vi "CRYUnflatten Stimulus.vi"(11 "Flatten Stimulus":string) -> (0 "Error?":bool=TRUE, 2 "Stimulus":T1={"StimulusType"="", "UseMLValArray"=[], "ML_axisArray"=[], "MLValLevelNameArray"=[], "Level(U)Array"=[1.0, 0.0, 0.0, 0.0, 0.0, 0.0, 0.26], "Start(Stop)FreqArray"=[20000.0, 20.0], "Start(Stop)AmpArray"=[0.5, 1.0], "StepResolutionArray"=[], "Unit_Array"=[], "DegValArray"=[], "DegUnitArray"=[], "Steps1"=19, "Cycle/step1(#)"=20, "Time/step1(s)"=0.01, "Transition1"=0.0, "SweepRate2"=1.0, "Freq3(Hz)"=0.0, "Steps3(#)"=19.0, "Cycles3(#)"=12, "StepSize3"=0.0, "wave time"="", "RMS_Value4"=0.0, "Peak_Value4"=0.0, "WavePath4"="", "RMS_unit4"="", "Peak_unit4"="", "wave Info"="", "dc_ctrl5_1"=0, "dc_ctrl5_2"=0, "dc_polar5"=0, "Max.Current"=0, "Steps5(#)"=19, "Time/Step5"=0.05, "Level5"=0.0, "StepsSize5Val"=0.0, "StepSize5Unit"="", "SweepType"=0, "Fixed/Ratio6"=0, "Transition6"=0.0, "Steps6(#)"=19.0, "Cycle/Steps6(#)"=12, "Time/Steps6(s)"=0.0, "Freq6(Hz)"=0.0, "Difference6(Hz)"=0.0, "Ratio6"="", "NoiseType7"=0, "Duration7(s)"=1.0, "MinFreq7(Hz)"=20000.0, "MaxFreq7(Hz)"=20.0, "MinFreq8(Hz)"=20000.0, "MaxFreq8(Hz)"=20.0, "FreqRounding8"=FALSE, "Duration8(s)"=1.0, "Tones8"=0.0, "RoundingVal8"=0.0, "ApplyEQ"=FALSE, "Duration(s)"=0.0, "CustomStimulusName "="", "Flatten Element Array"=[], "sine waves"=[], "Channel Out"=0, "RatioVal6"=0.0, "TabCtrl6"=enum."Master Tone", "Signal Type Name"="", "Help"="", "Channel Sel"=19, "V on DUT"=FALSE, "Output Imp"=6300.0, "Nominal Imp"=100.0} {"Nominal Imp" format="%.2p"; "Output Imp" format="%.2p"; "sine waves"."cycles" format="%.2f"; "sine waves"."ampl" format="%.2f"; "sine waves"."freq" format="%.2f"}, 3 "Header info":T2={"Data type"="Data            ", "Version"=1, "Dimensions"=0})   [LabVIEW 2013]
uses:
  Typedef Control/CRYStimulus Cluster.ctl
panel:
  # "(1,2,3,4,6_1,6_2,7,8)"
  # "(1,2,3,4,6_1,6_2,7,8)"
  # "(1,2,3,4,6_1,6_2,7,8)"
  # "(1,2,4,6_1,6_2,7,8)"
  # "(1,2,6)"
  # "(3,5)"
  # "(1,6,8)"
  # "(1,2,4,6_1,6_2,7,8)"
  # "(1,2,3,4,6_1,6_2,7,8)"
  # "(1,2,3,4,6_1,6_2,7,8)"
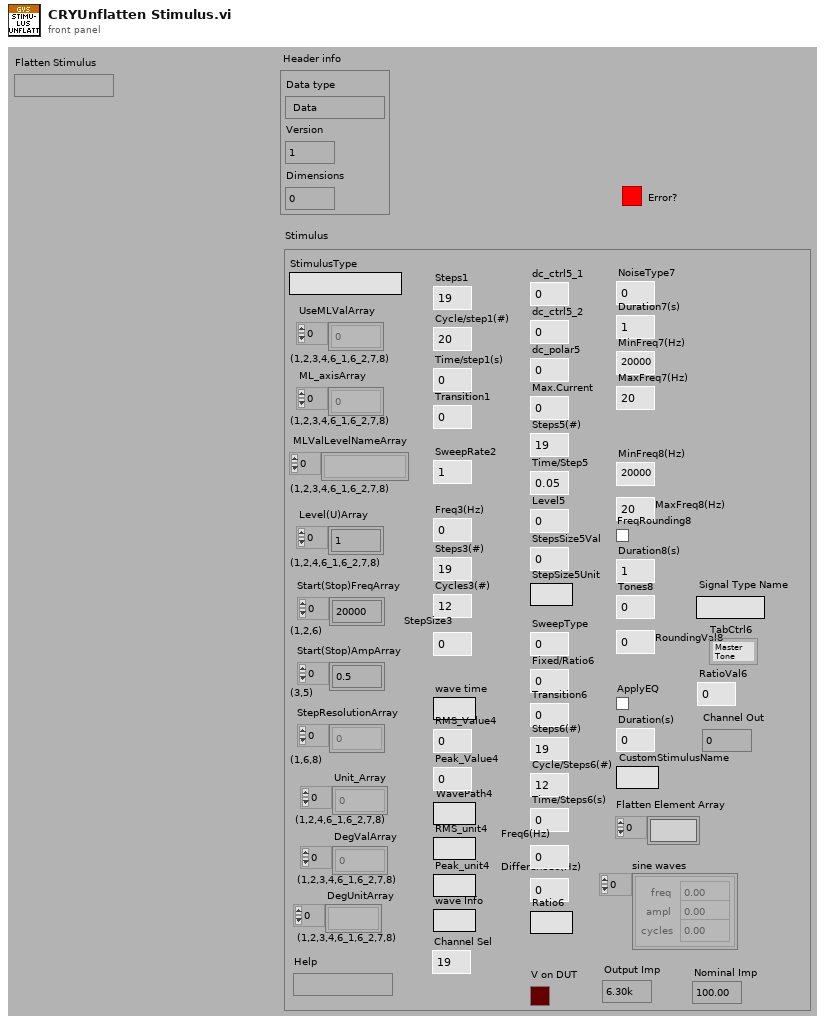
[diagram p1: front panel]
types:
  T1 = typedef "CRYStimulus Cluster.ctl" = cluster{"StimulusType":string, "UseMLValArray":u16[], "ML_axisArray":u16[], "MLValLevelNameArray":string[], "Level(U)Array":dbl[], "Start(Stop)FreqArray":dbl[], "Start(Stop)AmpArray":dbl[], "StepResolutionArray":u16[], "Unit_Array":u16[], "DegValArray":dbl[], "DegUnitArray":string[], "Steps1":i32, "Cycle/step1(#)":u32, "Time/step1(s)":dbl, "Transition1":dbl, "SweepRate2":dbl, "Freq3(Hz)":dbl, "Steps3(#)":dbl, "Cycles3(#)":u32, "StepSize3":dbl, "wave time":string, "RMS_Value4":dbl, "Peak_Value4":dbl, "WavePath4":string, "RMS_unit4":string, "Peak_unit4":string, "wave Info":string, "dc_ctrl5_1":u16, "dc_ctrl5_2":u16, "dc_polar5":u16, "Max.Current":u16, "Steps5(#)":u32, "Time/Step5":dbl, "Level5":dbl, "StepsSize5Val":dbl, "StepSize5Unit":string, "SweepType":u16, "Fixed/Ratio6":u16, "Transition6":dbl, "Steps6(#)":dbl, "Cycle/Steps6(#)":u32, "Time/Steps6(s)":dbl, "Freq6(Hz)":dbl, "Difference6(Hz)":dbl, "Ratio6":string, "NoiseType7":u16, "Duration7(s)":dbl, "MinFreq7(Hz)":dbl, "MaxFreq7(Hz)":dbl, "MinFreq8(Hz)":dbl, "MaxFreq8(Hz)":dbl, "FreqRounding8":bool, "Duration8(s)":dbl, "Tones8":dbl, "RoundingVal8":dbl, "ApplyEQ":bool, "Duration(s)":dbl, "CustomStimulusName ":string, "Flatten Element Array":string[], "sine waves":cluster{"freq":dbl, "ampl":dbl, "cycles":dbl}[], "Channel Out":i32, "RatioVal6":dbl, "TabCtrl6":enum32{"Master Tone", "Slave Tone"}, "Signal Type Name":string, "Help":string, "Channel Sel":u16, "V on DUT":bool, "Output Imp":dbl, "Nominal Imp":dbl}
  T2 = cluster{"Data type":string, "Version":u16, "Dimensions":u8}
  T3 = cluster{"unsigned byte array[0]":u8, "unsigned byte array[1]":u8, "unsigned byte array[2]":u8}
  T4 = cluster{"StimulusType":string, "UseMLValArray":u16[], "ML_axisArray":u16[], "MLValLevelNameArray":string[], "Level(U)Array":dbl[], "Start(Stop)FreqArray":dbl[], "Start(Stop)AmpArray":dbl[], "StepResolutionArray":string[], "Unit_Array":string[], "DegValArray":dbl[], "DegUnitArray":string[], "Steps1":i32, "Cycle/step1(#)":u32, "Time/step1(s)":dbl, "Transition1":dbl, "SweepRate2":dbl, "Freq3(Hz)":dbl, "Steps3(#)":dbl, "Cycles3(#)":u32, "StepSize3":dbl, "wave time":string, "RMS_Value4":dbl, "Peak_Value4":dbl, "WavePath4":string, "RMS_unit4":string, "Peak_unit4":string, "wave Info":string, "dc_ctrl5_1":u16, "dc_ctrl5_2":u16, "dc_polar5":u16, "Max.Current":u16, "Steps5(#)":u32, "Time/Step5":dbl, "Level5":dbl, "StepsSize5Val":dbl, "StepSize5Unit":string, "SweepType":u16, "Fixed/Ratio6":u16, "Transition6":dbl, "Steps6(#)":dbl, "Cycle/Steps6(#)":u32, "Time/Steps6(s)":dbl, "Freq6(Hz)":dbl, "Difference6(Hz)":dbl, "Ratio6":string, "NoiseType7":u16, "Duration7(s)":dbl, "MinFreq7(Hz)":dbl, "MaxFreq7(Hz)":dbl, "MinFreq8(Hz)":dbl, "MaxFreq8(Hz)":dbl, "FreqRounding8":bool, "Duration8(s)":dbl, "Tones8":dbl, "RoundingVal8":dbl, "ApplyEQ":bool, "Duration(s)":dbl, "CustomStimulusName ":string, "Flatten Element Array":string[], "sine waves":cluster{"freq":dbl, "ampl":dbl, "cycles":dbl}[], "Channel In":i32, "RatioVal6":dbl, "TabCtrl6":enum32{"Master Tone", "Slave Tone"}, "Channel Name":string}
  T5 = cluster{"StimulusType":string, "UseMLValArray":u16[], "ML_axisArray":u16[], "MLValLevelNameArray":string[], "Level(U)Array":dbl[], "Start(Stop)FreqArray":dbl[], "Start(Stop)AmpArray":dbl[], "StepResolutionArray":u16[], "Unit_Array":u16[], "DegValArray":dbl[], "DegUnitArray":string[], "Steps1":i32, "Cycle/step1(#)":u32, "Time/step1(s)":dbl, "Transition1":dbl, "SweepRate2":dbl, "Freq3(Hz)":dbl, "Steps3(#)":dbl, "Cycles3(#)":u32, "StepSize3":dbl, "wave time":string, "RMS_Value4":dbl, "Peak_Value4":dbl, "WavePath4":string, "RMS_unit4":string, "Peak_unit4":string, "wave Info":string, "dc_ctrl5_1":u16, "dc_ctrl5_2":u16, "dc_polar5":u16, "Max.Current":u16, "Steps5(#)":u32, "Time/Step5":dbl, "Level5":dbl, "StepsSize5Val":dbl, "StepSize5Unit":string, "SweepType":u16, "Fixed/Ratio6":u16, "Transition6":dbl, "Steps6(#)":dbl, "Cycle/Steps6(#)":u32, "Time/Steps6(s)":dbl, "Freq6(Hz)":dbl, "Difference6(Hz)":dbl, "Ratio6":string, "NoiseType7":u16, "Duration7(s)":dbl, "MinFreq7(Hz)":dbl, "MaxFreq7(Hz)":dbl, "MinFreq8(Hz)":dbl, "MaxFreq8(Hz)":dbl, "FreqRounding8":bool, "Duration8(s)":dbl, "Tones8":dbl, "RoundingVal8":dbl, "ApplyEQ":bool, "Duration(s)":dbl, "CustomStimulusName ":string, "Flatten Element Array":string[], "sine waves":cluster{"freq":dbl, "ampl":dbl, "cycles":dbl}[], "Channel In":i32, "RatioVal6":dbl, "TabCtrl6":enum32{"Master Tone", "Slave Tone"}, "Channel Name":string}
  T6 = cluster{"StimulusType":string, "UseMLValArray":u16[], "ML_axisArray":u16[], "MLValLevelNameArray":string[], "Level(U)Array":dbl[], "Start(Stop)FreqArray":dbl[], "Start(Stop)AmpArray":dbl[], "StepResolutionArray":u16[], "Unit_Array":u16[], "DegValArray":dbl[], "DegUnitArray":string[], "Steps1":i32, "Cycle/step1(#)":u32, "Time/step1(s)":dbl, "Transition1":dbl, "SweepRate2":dbl, "Freq3(Hz)":dbl, "Steps3(#)":dbl, "Cycles3(#)":u32, "StepSize3":dbl, "wave time":string, "RMS_Value4":dbl, "Peak_Value4":dbl, "WavePath4":string, "RMS_unit4":string, "Peak_unit4":string, "wave Info":string, "dc_ctrl5_1":u16, "dc_ctrl5_2":u16, "dc_polar5":u16, "Max.Current":u16, "Steps5(#)":u32, "Time/Step5":dbl, "Level5":dbl, "StepsSize5Val":dbl, "StepSize5Unit":string, "SweepType":u16, "Fixed/Ratio6":u16, "Transition6":dbl, "Steps6(#)":dbl, "Cycle/Steps6(#)":u32, "Time/Steps6(s)":dbl, "Freq6(Hz)":dbl, "Difference6(Hz)":dbl, "Ratio6":string, "NoiseType7":u16, "Duration7(s)":dbl, "MinFreq7(Hz)":dbl, "MaxFreq7(Hz)":dbl, "MinFreq8(Hz)":dbl, "MaxFreq8(Hz)":dbl, "FreqRounding8":bool, "Duration8(s)":dbl, "Tones8":dbl, "RoundingVal8":dbl, "ApplyEQ":bool, "Duration(s)":dbl, "CustomStimulusName ":string, "Flatten Element Array":string[], "sine waves":cluster{"freq":dbl, "ampl":dbl, "cycles":dbl}[], "Channel In":i32, "RatioVal6":dbl, "TabCtrl6":enum32{"Master Tone", "Slave Tone"}, "Channel Name":string, "Help":string}
  T7 = cluster{"StimulusType":string, "UseMLValArray":u16[], "ML_axisArray":u16[], "MLValLevelNameArray":string[], "Level(U)Array":dbl[], "Start(Stop)FreqArray":dbl[], "Start(Stop)AmpArray":dbl[], "StepResolutionArray":u16[], "Unit_Array":u16[], "DegValArray":dbl[], "DegUnitArray":string[], "Steps1":i32, "Cycle/step1(#)":u32, "Time/step1(s)":dbl, "Transition1":dbl, "SweepRate2":dbl, "Freq3(Hz)":dbl, "Steps3(#)":dbl, "Cycles3(#)":u32, "StepSize3":dbl, "wave time":string, "RMS_Value4":dbl, "Peak_Value4":dbl, "WavePath4":string, "RMS_unit4":string, "Peak_unit4":string, "wave Info":string, "dc_ctrl5_1":u16, "dc_ctrl5_2":u16, "dc_polar5":u16, "Max.Current":u16, "Steps5(#)":u32, "Time/Step5":dbl, "Level5":dbl, "StepsSize5Val":dbl, "StepSize5Unit":string, "SweepType":u16, "Fixed/Ratio6":u16, "Transition6":dbl, "Steps6(#)":dbl, "Cycle/Steps6(#)":u32, "Time/Steps6(s)":dbl, "Freq6(Hz)":dbl, "Difference6(Hz)":dbl, "Ratio6":string, "NoiseType7":u16, "Duration7(s)":dbl, "MinFreq7(Hz)":dbl, "MaxFreq7(Hz)":dbl, "MinFreq8(Hz)":dbl, "MaxFreq8(Hz)":dbl, "FreqRounding8":bool, "Duration8(s)":dbl, "Tones8":dbl, "RoundingVal8":dbl, "ApplyEQ":bool, "Duration(s)":dbl, "CustomStimulusName ":string, "Flatten Element Array":string[], "sine waves":cluster{"freq":dbl, "ampl":dbl, "cycles":dbl}[], "Channel Out":i32, "RatioVal6":dbl, "TabCtrl6":enum32{"Master Tone", "Slave Tone"}, "Signal Type Name":string, "Help":string, "Channel Sel":u16}
  T8 = cluster{"substring":string, u16, "unsigned byte array[2]":u8}
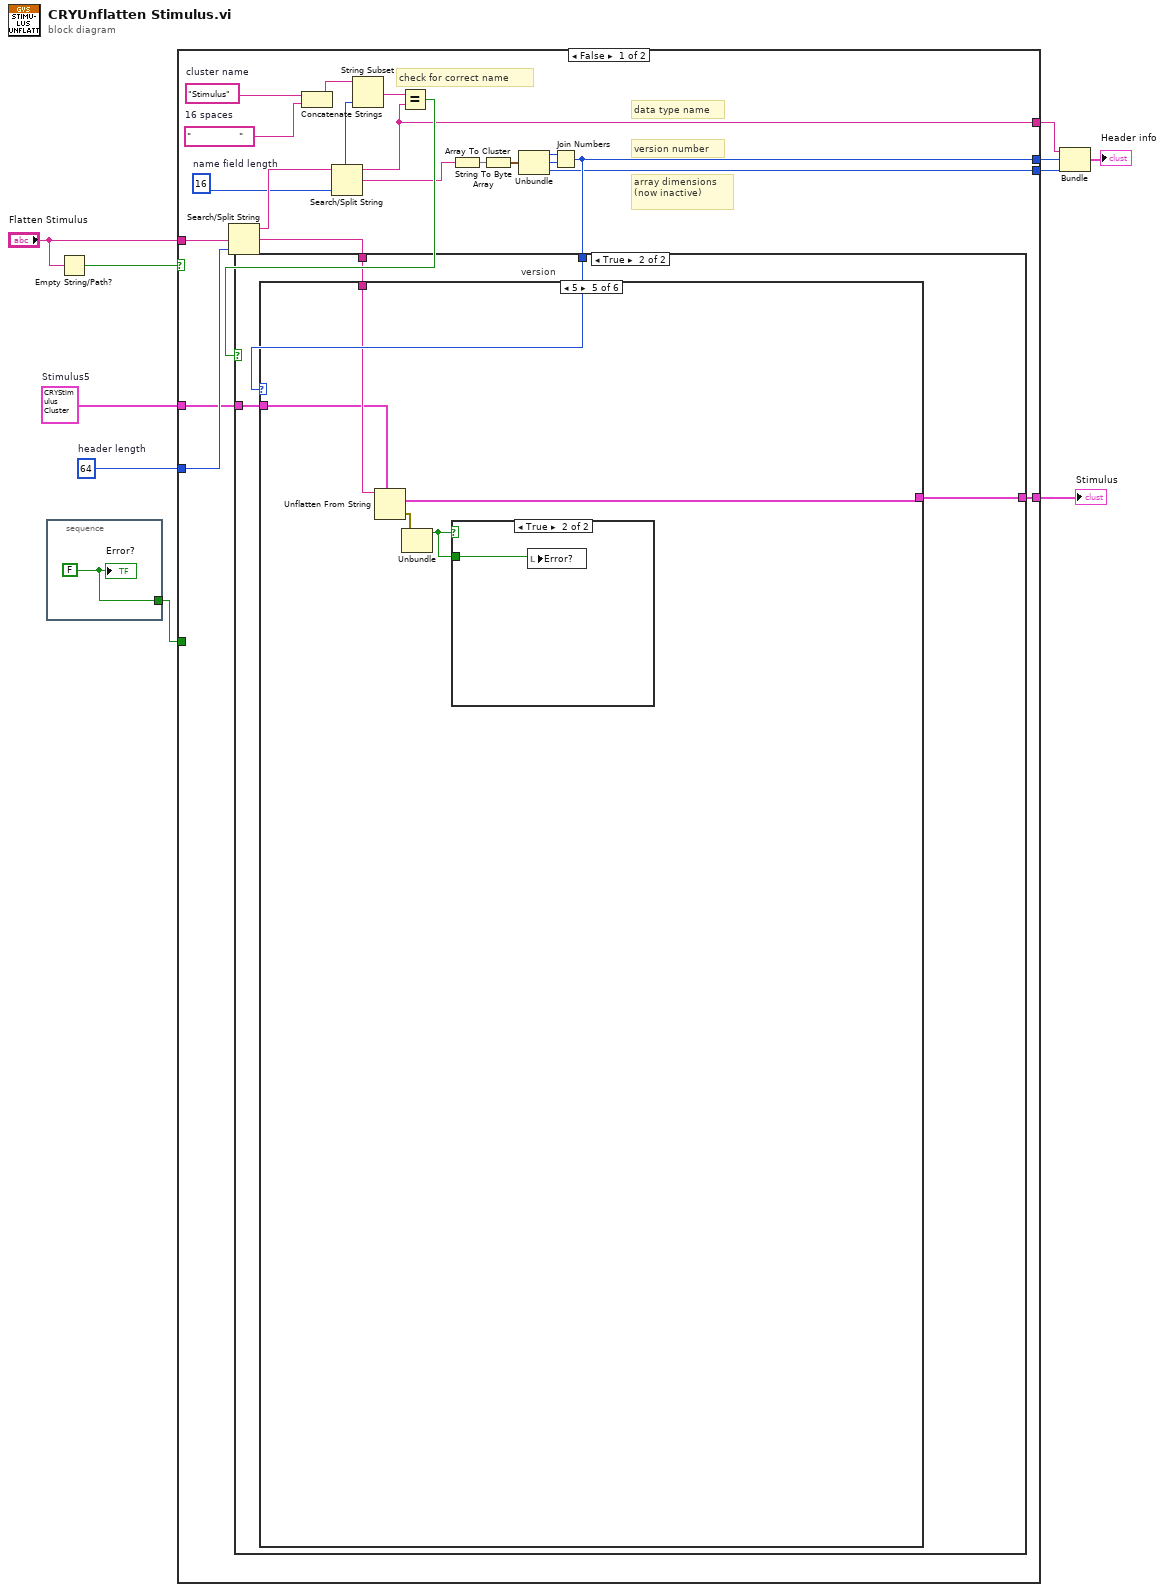
[diagram p0: block diagram]
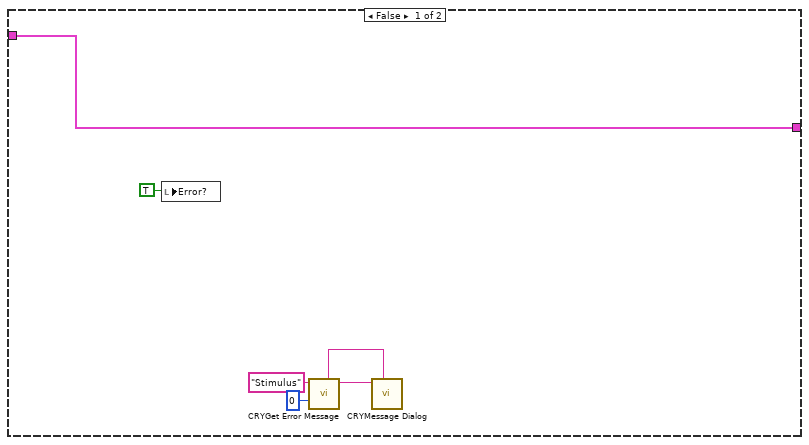
[diagram p2: hidden frame]
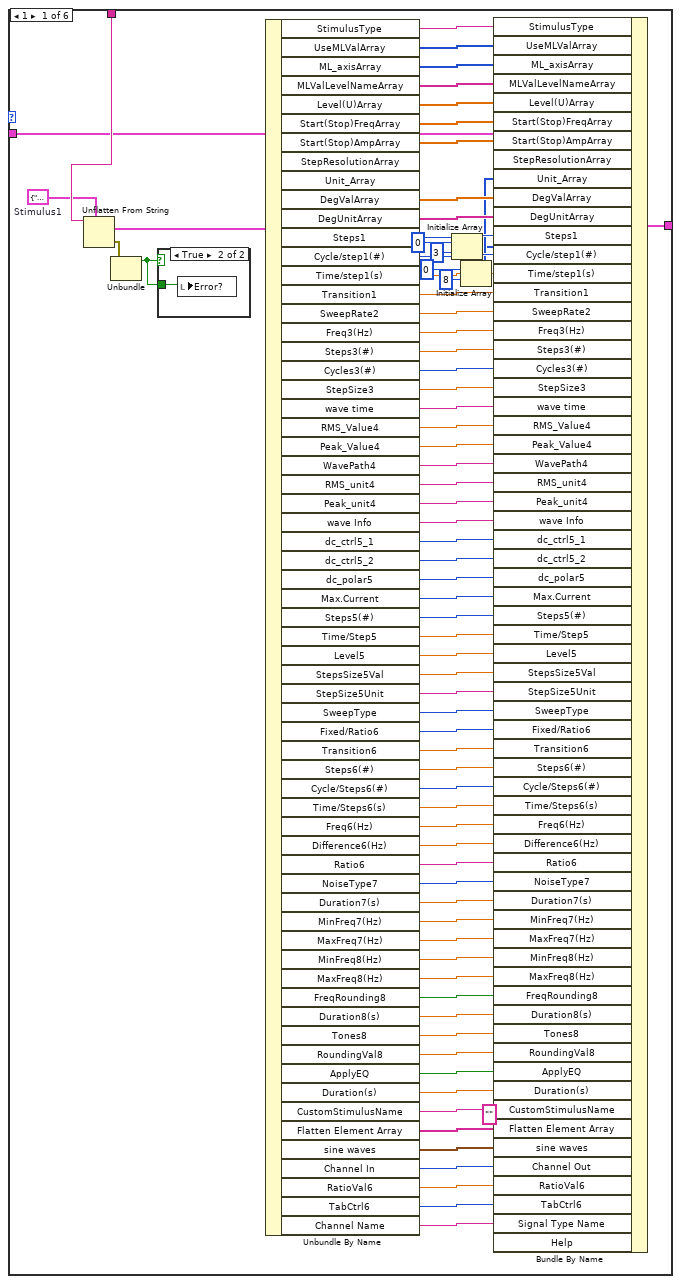
[diagram p3: hidden frame]
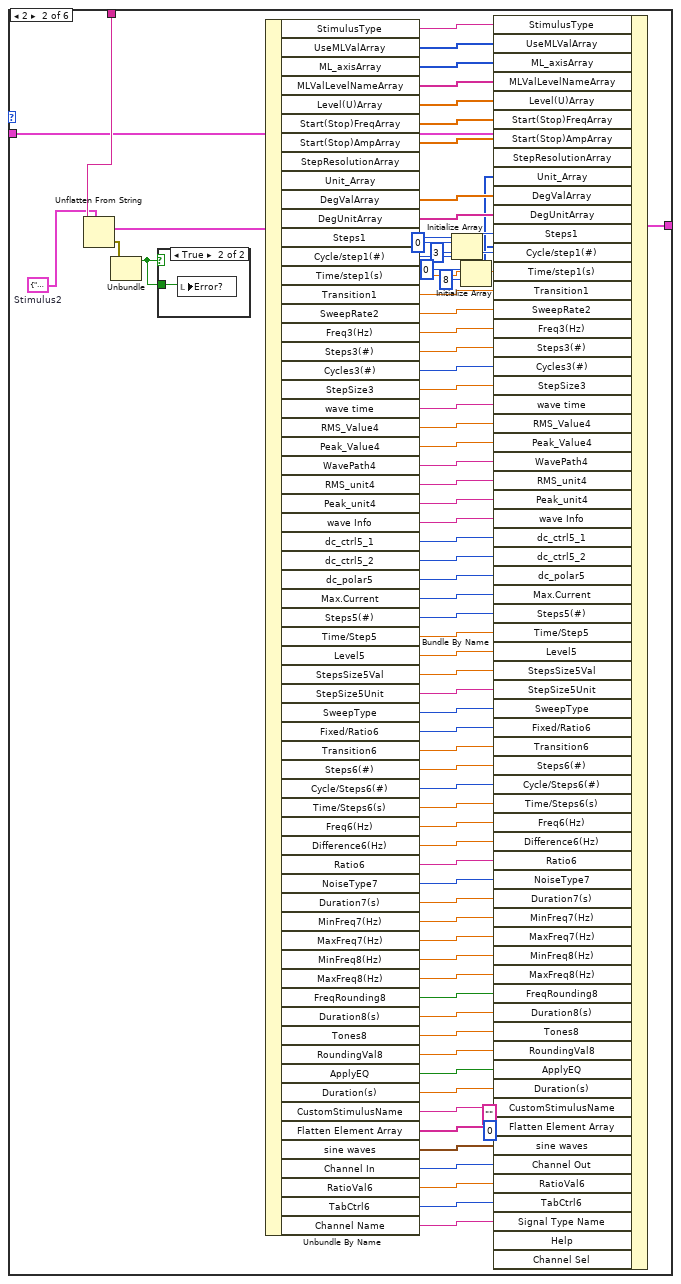
[diagram p5: hidden frame]
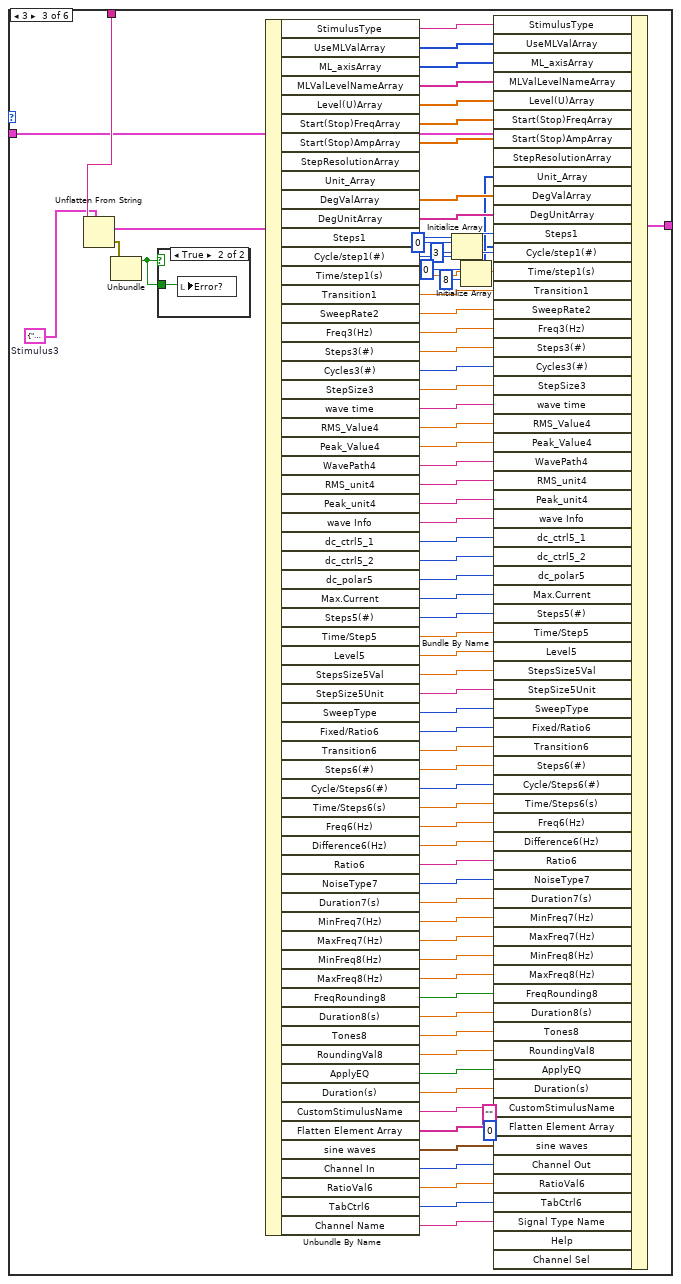
[diagram p7: hidden frame]
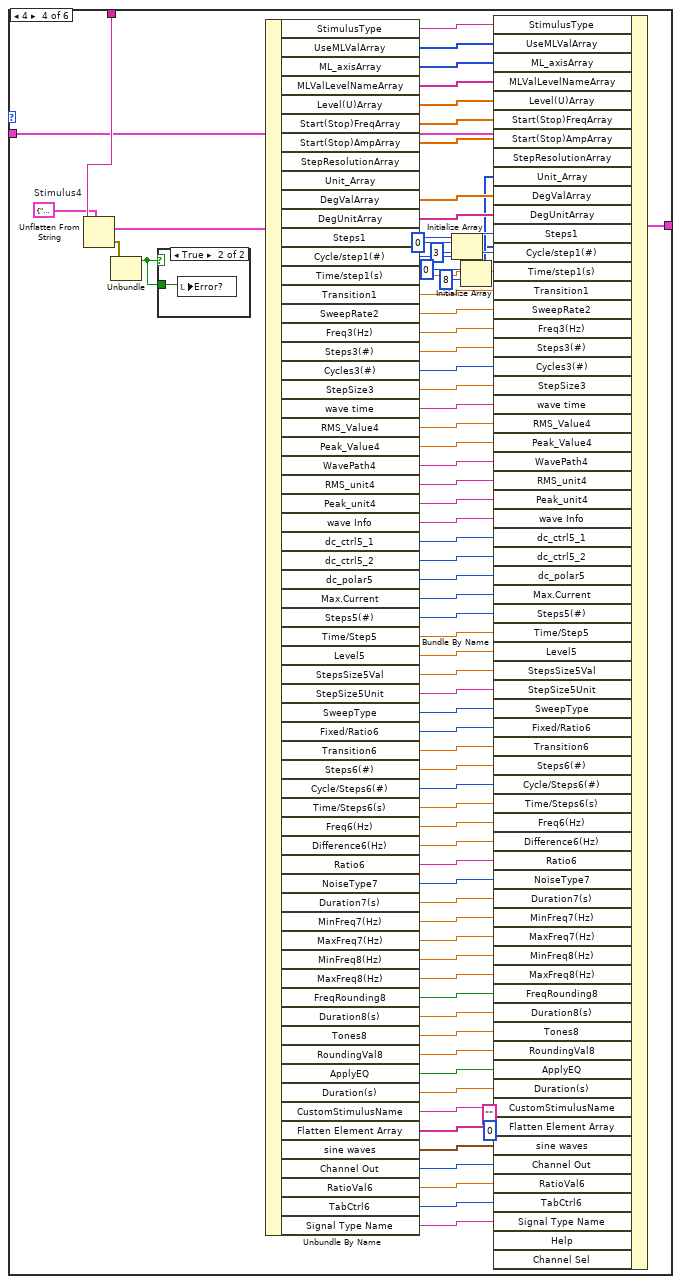
[diagram p9: hidden frame]
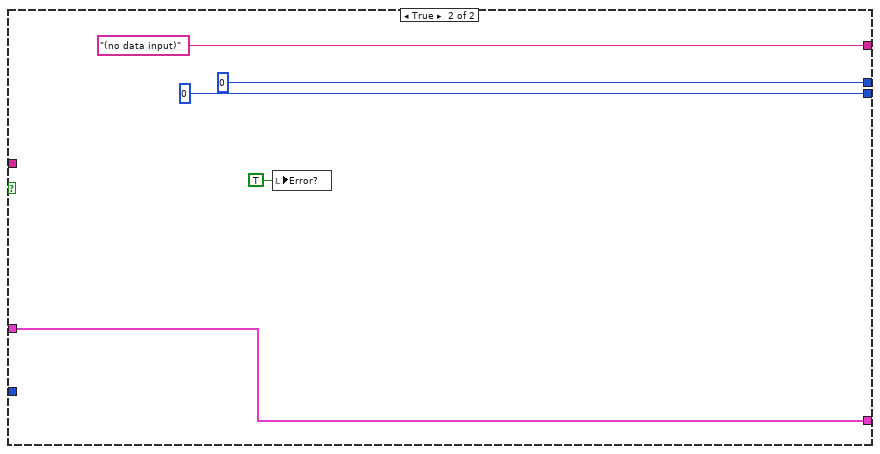
[diagram p13: hidden frame]
diagram:
  w1 = T1 {"StimulusType"="", "UseMLValArray"=[], "ML_axisArray"=[], "MLValLevelNameArray"=[], "Level(U)Array"=[], "Start(Stop)FreqArray"=[], "Start(Stop)AmpArray"=[], "StepResolutionArray"=[], "Unit_Array"=[], "DegValArray"=[], "DegUnitArray"=[], "Steps1"=0, "Cycle/step1(#)"=0, "Time/step1(s)"=0.0, "Transition1"=0.0, "SweepRate2"=0.0, "Freq3(Hz)"=0.0, "Steps3(#)"=0.0, "Cycles3(#)"=0, "StepSize3"=0.0, "wave time"="", "RMS_Value4"=0.0, "Peak_Value4"=0.0, "WavePath4"="", "RMS_unit4"="", "Peak_unit4"="", "wave Info"="", "dc_ctrl5_1"=0, "dc_ctrl5_2"=0, "dc_polar5"=0, "Max.Current"=0, "Steps5(#)"=0, "Time/Step5"=0.0, "Level5"=0.0, "StepsSize5Val"=0.0, "StepSize5Unit"="", "SweepType"=0, "Fixed/Ratio6"=0, "Transition6"=0.0, "Steps6(#)"=0.0, "Cycle/Steps6(#)"=0, "Time/Steps6(s)"=0.0, "Freq6(Hz)"=0.0, "Difference6(Hz)"=0.0, "Ratio6"="", "NoiseType7"=0, "Duration7(s)"=0.0, "MinFreq7(Hz)"=0.0, "MaxFreq7(Hz)"=0.0, "MinFreq8(Hz)"=0.0, "MaxFreq8(Hz)"=0.0, "FreqRounding8"=FALSE, "Duration8(s)"=0.0, "Tones8"=0.0, "RoundingVal8"=0.0, "ApplyEQ"=FALSE, "Duration(s)"=0.0, "CustomStimulusName "="", "Flatten Element Array"=[], "sine waves"=[], "Channel Out"=0, "RatioVal6"=0.0, "TabCtrl6"=enum."Master Tone", "Signal Type Name"="", "Help"="", "Channel Sel"=0, "V on DUT"=FALSE, "Output Imp"=0.0, "Nominal Imp"=0.0}  # Stimulus5
  w8 = 64  # header length
  n1 = stacked-sequence {
    tunnel: [w11] -> w3
    frame #0 {
      w11 = FALSE
      "Error?" <- w11
    }
  }
  n2 = Empty String/Path?(string/path="Flatten Stimulus") -> (empty?=w9:bool)
  n3 = case shown="False" w9 {
    tunnel: "Flatten Stimulus" -> [w31 _]
    tunnel: w8 -> [w25 _]
    tunnel: [w22 u16 0] -> w6
    tunnel: [w14 u8 0] -> w7
    tunnel: [w15 "(no data input)" ("substring")] -> w5
    tunnel: w3 -> [_ _]
    tunnel: [w13 w360] -> w2
    tunnel: w1 -> [w12 w360]
    frame False {
      w19 = "                "  # 16 spaces
      w20 = "Stimulus"  # cluster name
      w17 = 16  # name field length
      # "check for correct name"
      # "array dimensions\n(now inactive)"
      # "version number"
      # "data type name"
      n4 = Search/Split String(string=w31, offset (0)=w25) -> (substring before match=w24:string, match + rest of string=w26:string)  [unwired: 2 out]
      n5 = Concatenate Strings(w20, w19) -> (w18:string)
      n6 = Search/Split String(string=w24, offset (0)=w17) -> (substring before match=w15:string, match + rest of string=w21:string)  [unwired: 2 out]
      n7 = String Subset(string=w18, length (rest)=w17) -> (substring=w16:string)  [unwired: 1 out]
      n8 = Equal?(x=w16, y=w15) -> (x = y?=w23:bool)
      n9 = String To Byte Array(string=w21) -> (unsigned byte array=w30:u8[])
      n10 = Array To Cluster(array=w30) -> (cluster=w29:T3)
      n11 = Unbundle(w29) -> ("unsigned byte array[0]"=w28:u8, "unsigned byte array[1]"=w27:u8, "unsigned byte array[2]"=w14:u8)
      n12 = Join Numbers(hi=w28, lo=w27) -> ((hi.lo)=w22:u16)
      n13 = case shown="True" w23 {
        tunnel: w26 -> [_ w41]
        tunnel: w22 -> [_ w40]
        tunnel: [w36 w39] -> w13
        tunnel: w12 -> [w36 w38]
        frame False {
          n14 = local write "Error?"(TRUE) -> ()
          n15 = call "CRYGet Error Message.vi"("Error No"=0, "Kind"="Stimulus") -> ("Message"=w33:string, "Window Title"=w32:string)  [unwired: 4 in, 4 out]
          n16 = call "CRYMessage Dialog.vi"("Window Title"=w32, "Message Content"=w33) -> ()  [unwired: 8 in, 2 out]
        }
        frame True {
          n17 = case "version" shown="5" w40 {
            tunnel: w41 -> [w117 w195 w273 w351 w357 _]
            tunnel: [w112 w190 w268 w346 w353 w359] -> w39
            tunnel: w38 -> [w114 w192 w270 w348 w354 w359]
            frame 1 {
              w43 = T4 {"StimulusType"="", "UseMLValArray"=[], "ML_axisArray"=[], "MLValLevelNameArray"=[], "Level(U)Array"=[], "Start(Stop)FreqArray"=[], "Start(Stop)AmpArray"=[], "StepResolutionArray"=[], "Unit_Array"=[], "DegValArray"=[], "DegUnitArray"=[], "Steps1"=0, "Cycle/step1(#)"=0, "Time/step1(s)"=0.0, "Transition1"=0.0, "SweepRate2"=0.0, "Freq3(Hz)"=0.0, "Steps3(#)"=0.0, "Cycles3(#)"=0, "StepSize3"=0.0, "wave time"="", "RMS_Value4"=0.0, "Peak_Value4"=0.0, "WavePath4"="", "RMS_unit4"="", "Peak_unit4"="", "wave Info"="", "dc_ctrl5_1"=0, "dc_ctrl5_2"=0, "dc_polar5"=0, "Max.Current"=0, "Steps5(#)"=0, "Time/Step5"=0.0, "Level5"=0.0, "StepsSize5Val"=0.0, "StepSize5Unit"="", "SweepType"=0, "Fixed/Ratio6"=0, "Transition6"=0.0, "Steps6(#)"=0.0, "Cycle/Steps6(#)"=0, "Time/Steps6(s)"=0.0, "Freq6(Hz)"=0.0, "Difference6(Hz)"=0.0, "Ratio6"="", "NoiseType7"=0, "Duration7(s)"=0.0, "MinFreq7(Hz)"=0.0, "MaxFreq7(Hz)"=0.0, "MinFreq8(Hz)"=0.0, "MaxFreq8(Hz)"=0.0, "FreqRounding8"=FALSE, "Duration8(s)"=0.0, "Tones8"=0.0, "RoundingVal8"=0.0, "ApplyEQ"=FALSE, "Duration(s)"=0.0, "CustomStimulusName "="", "Flatten Element Array"=[], "sine waves"=[], "Channel In"=0, "RatioVal6"=0.0, "TabCtrl6"=enum."Master Tone", "Channel Name"=""}  # Stimulus1
              n18 = Unflatten From String(type=w43, binary string=w117) -> (value=w113:T4, error out=w115:errorcluster)  [unwired: 1 in, 3 out]
              n19 = Unbundle(w115) -> ("status"=w116:bool)  [unwired: 2 out]
              n20 = case shown="True" w116 {
                tunnel: w116 -> [_ w118]
                frame False {
                }
                frame True {
                  n21 = local write "Error?"(w118) -> ()
                }
              }
              n22 = Unbundle By Name(w113) -> ("StimulusType"=w111:string, "UseMLValArray"=w110:u16[], "ML_axisArray"=w109:u16[], "MLValLevelNameArray"=w105:string[], "Level(U)Array"=w106:dbl[], "Start(Stop)FreqArray"=w107:dbl[], "Start(Stop)AmpArray"=w108:dbl[], "DegValArray"=w104:dbl[], "DegUnitArray"=w103:string[], "Steps1"=w102:i32, "Cycle/step1(#)"=w101:u32, "Time/step1(s)"=w100:dbl, "Transition1"=w99:dbl, "SweepRate2"=w98:dbl, "Freq3(Hz)"=w97:dbl, "Steps3(#)"=w96:dbl, "Cycles3(#)"=w95:u32, "StepSize3"=w94:dbl, "wave time"=w93:string, "RMS_Value4"=w92:dbl, "Peak_Value4"=w91:dbl, "WavePath4"=w90:string, "RMS_unit4"=w89:string, "Peak_unit4"=w88:string, "wave Info"=w87:string, "dc_ctrl5_1"=w86:u16, "dc_ctrl5_2"=w85:u16, "dc_polar5"=w84:u16, "Max.Current"=w83:u16, "Steps5(#)"=w82:u32, "Time/Step5"=w81:dbl, "Level5"=w80:dbl, "StepsSize5Val"=w79:dbl, "StepSize5Unit"=w78:string, "SweepType"=w77:u16, "Fixed/Ratio6"=w76:u16, "Transition6"=w75:dbl, "Steps6(#)"=w74:dbl, "Cycle/Steps6(#)"=w73:u32, "Time/Steps6(s)"=w72:dbl, "Freq6(Hz)"=w71:dbl, "Difference6(Hz)"=w70:dbl, "Ratio6"=w69:string, "NoiseType7"=w68:u16, "Duration7(s)"=w67:dbl, "MinFreq7(Hz)"=w66:dbl, "MaxFreq7(Hz)"=w65:dbl, "MinFreq8(Hz)"=w64:dbl, "MaxFreq8(Hz)"=w63:dbl, "FreqRounding8"=w62:bool, "Duration8(s)"=w61:dbl, "Tones8"=w60:dbl, "RoundingVal8"=w59:dbl, "ApplyEQ"=w58:bool, "Duration(s)"=w57:dbl, "CustomStimulusName"=w56:string, "Flatten Element Array"=w55:string[], "sine waves"=w54:cluster{"freq":dbl, "ampl":dbl, "cycles":dbl}[], "Channel In"=w53:i32, "RatioVal6"=w52:dbl, "TabCtrl6"=w51:enum32{"Master Tone", "Slave Tone"}, "Channel Name"=w50:string)  [unwired: 2 out]
              n23 = Initialize Array(u16 0 ("Unit"), 3 ("dimension size")) -> (w44:u16[])
              n24 = Initialize Array(u16 0 ("Unit"), 8 ("dimension size")) -> (w47:u16[])
              n25 = Bundle By Name(cluster=w114, "StimulusType"=w111, "UseMLValArray"=w110, "ML_axisArray"=w109, "MLValLevelNameArray"=w105, "Level(U)Array"=w106, "Start(Stop)FreqArray"=w107, "Start(Stop)AmpArray"=w108, "StepResolutionArray"=w44, "Unit_Array"=w47, "DegValArray"=w104, "DegUnitArray"=w103, "Steps1"=w102, "Cycle/step1(#)"=w101, "Time/step1(s)"=w100, "Transition1"=w99, "SweepRate2"=w98, "Freq3(Hz)"=w97, "Steps3(#)"=w96, "Cycles3(#)"=w95, "StepSize3"=w94, "wave time"=w93, "RMS_Value4"=w92, "Peak_Value4"=w91, "WavePath4"=w90, "RMS_unit4"=w89, "Peak_unit4"=w88, "wave Info"=w87, "dc_ctrl5_1"=w86, "dc_ctrl5_2"=w85, "dc_polar5"=w84, "Max.Current"=w83, "Steps5(#)"=w82, "Time/Step5"=w81, "Level5"=w80, "StepsSize5Val"=w79, "StepSize5Unit"=w78, "SweepType"=w77, "Fixed/Ratio6"=w76, "Transition6"=w75, "Steps6(#)"=w74, "Cycle/Steps6(#)"=w73, "Time/Steps6(s)"=w72, "Freq6(Hz)"=w71, "Difference6(Hz)"=w70, "Ratio6"=w69, "NoiseType7"=w68, "Duration7(s)"=w67, "MinFreq7(Hz)"=w66, "MaxFreq7(Hz)"=w65, "MinFreq8(Hz)"=w64, "MaxFreq8(Hz)"=w63, "FreqRounding8"=w62, "Duration8(s)"=w61, "Tones8"=w60, "RoundingVal8"=w59, "ApplyEQ"=w58, "Duration(s)"=w57, "CustomStimulusName"=w56, "Flatten Element Array"=w55, "sine waves"=w54, "Channel Out"=w53, "RatioVal6"=w52, "TabCtrl6"=w51, "Signal Type Name"=w50, "Help"="") -> (w112:T1)
            }
            frame 2 {
              w121 = T5 {"StimulusType"="", "UseMLValArray"=[], "ML_axisArray"=[], "MLValLevelNameArray"=[], "Level(U)Array"=[], "Start(Stop)FreqArray"=[], "Start(Stop)AmpArray"=[], "StepResolutionArray"=[], "Unit_Array"=[], "DegValArray"=[], "DegUnitArray"=[], "Steps1"=0, "Cycle/step1(#)"=0, "Time/step1(s)"=0.0, "Transition1"=0.0, "SweepRate2"=0.0, "Freq3(Hz)"=0.0, "Steps3(#)"=0.0, "Cycles3(#)"=0, "StepSize3"=0.0, "wave time"="", "RMS_Value4"=0.0, "Peak_Value4"=0.0, "WavePath4"="", "RMS_unit4"="", "Peak_unit4"="", "wave Info"="", "dc_ctrl5_1"=0, "dc_ctrl5_2"=0, "dc_polar5"=0, "Max.Current"=0, "Steps5(#)"=0, "Time/Step5"=0.0, "Level5"=0.0, "StepsSize5Val"=0.0, "StepSize5Unit"="", "SweepType"=0, "Fixed/Ratio6"=0, "Transition6"=0.0, "Steps6(#)"=0.0, "Cycle/Steps6(#)"=0, "Time/Steps6(s)"=0.0, "Freq6(Hz)"=0.0, "Difference6(Hz)"=0.0, "Ratio6"="", "NoiseType7"=0, "Duration7(s)"=0.0, "MinFreq7(Hz)"=0.0, "MaxFreq7(Hz)"=0.0, "MinFreq8(Hz)"=0.0, "MaxFreq8(Hz)"=0.0, "FreqRounding8"=FALSE, "Duration8(s)"=0.0, "Tones8"=0.0, "RoundingVal8"=0.0, "ApplyEQ"=FALSE, "Duration(s)"=0.0, "CustomStimulusName "="", "Flatten Element Array"=[], "sine waves"=[], "Channel In"=0, "RatioVal6"=0.0, "TabCtrl6"=enum."Master Tone", "Channel Name"=""}  # Stimulus2
              n26 = Unflatten From String(type=w121, binary string=w195) -> (value=w191:T5, error out=w193:errorcluster)  [unwired: 1 in, 3 out]
              n27 = Unbundle(w193) -> ("status"=w194:bool)  [unwired: 2 out]
              n28 = case shown="True" w194 {
                tunnel: w194 -> [_ w196]
                frame False {
                }
                frame True {
                  n29 = local write "Error?"(w196) -> ()
                }
              }
              n30 = Unbundle By Name(w191) -> ("StimulusType"=w189:string, "UseMLValArray"=w188:u16[], "ML_axisArray"=w187:u16[], "MLValLevelNameArray"=w183:string[], "Level(U)Array"=w184:dbl[], "Start(Stop)FreqArray"=w185:dbl[], "Start(Stop)AmpArray"=w186:dbl[], "DegValArray"=w182:dbl[], "DegUnitArray"=w181:string[], "Steps1"=w180:i32, "Cycle/step1(#)"=w179:u32, "Time/step1(s)"=w178:dbl, "Transition1"=w177:dbl, "SweepRate2"=w176:dbl, "Freq3(Hz)"=w175:dbl, "Steps3(#)"=w174:dbl, "Cycles3(#)"=w173:u32, "StepSize3"=w172:dbl, "wave time"=w171:string, "RMS_Value4"=w170:dbl, "Peak_Value4"=w169:dbl, "WavePath4"=w168:string, "RMS_unit4"=w167:string, "Peak_unit4"=w166:string, "wave Info"=w165:string, "dc_ctrl5_1"=w164:u16, "dc_ctrl5_2"=w163:u16, "dc_polar5"=w162:u16, "Max.Current"=w161:u16, "Steps5(#)"=w160:u32, "Time/Step5"=w159:dbl, "Level5"=w158:dbl, "StepsSize5Val"=w157:dbl, "StepSize5Unit"=w156:string, "SweepType"=w155:u16, "Fixed/Ratio6"=w154:u16, "Transition6"=w153:dbl, "Steps6(#)"=w152:dbl, "Cycle/Steps6(#)"=w151:u32, "Time/Steps6(s)"=w150:dbl, "Freq6(Hz)"=w149:dbl, "Difference6(Hz)"=w148:dbl, "Ratio6"=w147:string, "NoiseType7"=w146:u16, "Duration7(s)"=w145:dbl, "MinFreq7(Hz)"=w144:dbl, "MaxFreq7(Hz)"=w143:dbl, "MinFreq8(Hz)"=w142:dbl, "MaxFreq8(Hz)"=w141:dbl, "FreqRounding8"=w140:bool, "Duration8(s)"=w139:dbl, "Tones8"=w138:dbl, "RoundingVal8"=w137:dbl, "ApplyEQ"=w136:bool, "Duration(s)"=w135:dbl, "CustomStimulusName"=w134:string, "Flatten Element Array"=w133:string[], "sine waves"=w132:cluster{"freq":dbl, "ampl":dbl, "cycles":dbl}[], "Channel In"=w131:i32, "RatioVal6"=w130:dbl, "TabCtrl6"=w129:enum32{"Master Tone", "Slave Tone"}, "Channel Name"=w128:string)  [unwired: 2 out]
              n31 = Initialize Array(u16 0 ("Unit"), 3 ("dimension size")) -> (w122:u16[])
              n32 = Initialize Array(u16 0 ("Unit"), 8 ("dimension size")) -> (w125:u16[])
              n33 = Bundle By Name(cluster=w192, "StimulusType"=w189, "UseMLValArray"=w188, "ML_axisArray"=w187, "MLValLevelNameArray"=w183, "Level(U)Array"=w184, "Start(Stop)FreqArray"=w185, "Start(Stop)AmpArray"=w186, "StepResolutionArray"=w122, "Unit_Array"=w125, "DegValArray"=w182, "DegUnitArray"=w181, "Steps1"=w180, "Cycle/step1(#)"=w179, "Time/step1(s)"=w178, "Transition1"=w177, "SweepRate2"=w176, "Freq3(Hz)"=w175, "Steps3(#)"=w174, "Cycles3(#)"=w173, "StepSize3"=w172, "wave time"=w171, "RMS_Value4"=w170, "Peak_Value4"=w169, "WavePath4"=w168, "RMS_unit4"=w167, "Peak_unit4"=w166, "wave Info"=w165, "dc_ctrl5_1"=w164, "dc_ctrl5_2"=w163, "dc_polar5"=w162, "Max.Current"=w161, "Steps5(#)"=w160, "Time/Step5"=w159, "Level5"=w158, "StepsSize5Val"=w157, "StepSize5Unit"=w156, "SweepType"=w155, "Fixed/Ratio6"=w154, "Transition6"=w153, "Steps6(#)"=w152, "Cycle/Steps6(#)"=w151, "Time/Steps6(s)"=w150, "Freq6(Hz)"=w149, "Difference6(Hz)"=w148, "Ratio6"=w147, "NoiseType7"=w146, "Duration7(s)"=w145, "MinFreq7(Hz)"=w144, "MaxFreq7(Hz)"=w143, "MinFreq8(Hz)"=w142, "MaxFreq8(Hz)"=w141, "FreqRounding8"=w140, "Duration8(s)"=w139, "Tones8"=w138, "RoundingVal8"=w137, "ApplyEQ"=w136, "Duration(s)"=w135, "CustomStimulusName"=w134, "Flatten Element Array"=w133, "sine waves"=w132, "Channel Out"=w131, "RatioVal6"=w130, "TabCtrl6"=w129, "Signal Type Name"=w128, "Help"="", "Channel Sel"=0 ("wave channel")) -> (w190:T1)
            }
            frame 3 {
              w198 = T6 {"StimulusType"="", "UseMLValArray"=[], "ML_axisArray"=[], "MLValLevelNameArray"=[], "Level(U)Array"=[], "Start(Stop)FreqArray"=[], "Start(Stop)AmpArray"=[], "StepResolutionArray"=[], "Unit_Array"=[], "DegValArray"=[], "DegUnitArray"=[], "Steps1"=0, "Cycle/step1(#)"=0, "Time/step1(s)"=0.0, "Transition1"=0.0, "SweepRate2"=0.0, "Freq3(Hz)"=0.0, "Steps3(#)"=0.0, "Cycles3(#)"=0, "StepSize3"=0.0, "wave time"="", "RMS_Value4"=0.0, "Peak_Value4"=0.0, "WavePath4"="", "RMS_unit4"="", "Peak_unit4"="", "wave Info"="", "dc_ctrl5_1"=0, "dc_ctrl5_2"=0, "dc_polar5"=0, "Max.Current"=0, "Steps5(#)"=0, "Time/Step5"=0.0, "Level5"=0.0, "StepsSize5Val"=0.0, "StepSize5Unit"="", "SweepType"=0, "Fixed/Ratio6"=0, "Transition6"=0.0, "Steps6(#)"=0.0, "Cycle/Steps6(#)"=0, "Time/Steps6(s)"=0.0, "Freq6(Hz)"=0.0, "Difference6(Hz)"=0.0, "Ratio6"="", "NoiseType7"=0, "Duration7(s)"=0.0, "MinFreq7(Hz)"=0.0, "MaxFreq7(Hz)"=0.0, "MinFreq8(Hz)"=0.0, "MaxFreq8(Hz)"=0.0, "FreqRounding8"=FALSE, "Duration8(s)"=0.0, "Tones8"=0.0, "RoundingVal8"=0.0, "ApplyEQ"=FALSE, "Duration(s)"=0.0, "CustomStimulusName "="", "Flatten Element Array"=[], "sine waves"=[], "Channel In"=0, "RatioVal6"=0.0, "TabCtrl6"=enum."Master Tone", "Channel Name"="", "Help"=""}  # Stimulus3
              n34 = Unflatten From String(type=w198, binary string=w273) -> (value=w269:T6, error out=w271:errorcluster)  [unwired: 1 in, 3 out]
              n35 = Unbundle(w271) -> ("status"=w272:bool)  [unwired: 2 out]
              n36 = case shown="True" w272 {
                tunnel: w272 -> [_ w274]
                frame False {
                }
                frame True {
                  n37 = local write "Error?"(w274) -> ()
                }
              }
              n38 = Unbundle By Name(w269) -> ("StimulusType"=w267:string, "UseMLValArray"=w266:u16[], "ML_axisArray"=w265:u16[], "MLValLevelNameArray"=w261:string[], "Level(U)Array"=w262:dbl[], "Start(Stop)FreqArray"=w263:dbl[], "Start(Stop)AmpArray"=w264:dbl[], "DegValArray"=w260:dbl[], "DegUnitArray"=w259:string[], "Steps1"=w258:i32, "Cycle/step1(#)"=w257:u32, "Time/step1(s)"=w256:dbl, "Transition1"=w255:dbl, "SweepRate2"=w254:dbl, "Freq3(Hz)"=w253:dbl, "Steps3(#)"=w252:dbl, "Cycles3(#)"=w251:u32, "StepSize3"=w250:dbl, "wave time"=w249:string, "RMS_Value4"=w248:dbl, "Peak_Value4"=w247:dbl, "WavePath4"=w246:string, "RMS_unit4"=w245:string, "Peak_unit4"=w244:string, "wave Info"=w243:string, "dc_ctrl5_1"=w242:u16, "dc_ctrl5_2"=w241:u16, "dc_polar5"=w240:u16, "Max.Current"=w239:u16, "Steps5(#)"=w238:u32, "Time/Step5"=w237:dbl, "Level5"=w236:dbl, "StepsSize5Val"=w235:dbl, "StepSize5Unit"=w234:string, "SweepType"=w233:u16, "Fixed/Ratio6"=w232:u16, "Transition6"=w231:dbl, "Steps6(#)"=w230:dbl, "Cycle/Steps6(#)"=w229:u32, "Time/Steps6(s)"=w228:dbl, "Freq6(Hz)"=w227:dbl, "Difference6(Hz)"=w226:dbl, "Ratio6"=w225:string, "NoiseType7"=w224:u16, "Duration7(s)"=w223:dbl, "MinFreq7(Hz)"=w222:dbl, "MaxFreq7(Hz)"=w221:dbl, "MinFreq8(Hz)"=w220:dbl, "MaxFreq8(Hz)"=w219:dbl, "FreqRounding8"=w218:bool, "Duration8(s)"=w217:dbl, "Tones8"=w216:dbl, "RoundingVal8"=w215:dbl, "ApplyEQ"=w214:bool, "Duration(s)"=w213:dbl, "CustomStimulusName"=w212:string, "Flatten Element Array"=w211:string[], "sine waves"=w210:cluster{"freq":dbl, "ampl":dbl, "cycles":dbl}[], "Channel In"=w209:i32, "RatioVal6"=w208:dbl, "TabCtrl6"=w207:enum32{"Master Tone", "Slave Tone"}, "Channel Name"=w206:string)  [unwired: 2 out]
              n39 = Initialize Array(u16 0 ("Unit"), 3 ("dimension size")) -> (w200:u16[])
              n40 = Initialize Array(u16 0 ("Unit"), 8 ("dimension size")) -> (w203:u16[])
              n41 = Bundle By Name(cluster=w270, "StimulusType"=w267, "UseMLValArray"=w266, "ML_axisArray"=w265, "MLValLevelNameArray"=w261, "Level(U)Array"=w262, "Start(Stop)FreqArray"=w263, "Start(Stop)AmpArray"=w264, "StepResolutionArray"=w200, "Unit_Array"=w203, "DegValArray"=w260, "DegUnitArray"=w259, "Steps1"=w258, "Cycle/step1(#)"=w257, "Time/step1(s)"=w256, "Transition1"=w255, "SweepRate2"=w254, "Freq3(Hz)"=w253, "Steps3(#)"=w252, "Cycles3(#)"=w251, "StepSize3"=w250, "wave time"=w249, "RMS_Value4"=w248, "Peak_Value4"=w247, "WavePath4"=w246, "RMS_unit4"=w245, "Peak_unit4"=w244, "wave Info"=w243, "dc_ctrl5_1"=w242, "dc_ctrl5_2"=w241, "dc_polar5"=w240, "Max.Current"=w239, "Steps5(#)"=w238, "Time/Step5"=w237, "Level5"=w236, "StepsSize5Val"=w235, "StepSize5Unit"=w234, "SweepType"=w233, "Fixed/Ratio6"=w232, "Transition6"=w231, "Steps6(#)"=w230, "Cycle/Steps6(#)"=w229, "Time/Steps6(s)"=w228, "Freq6(Hz)"=w227, "Difference6(Hz)"=w226, "Ratio6"=w225, "NoiseType7"=w224, "Duration7(s)"=w223, "MinFreq7(Hz)"=w222, "MaxFreq7(Hz)"=w221, "MinFreq8(Hz)"=w220, "MaxFreq8(Hz)"=w219, "FreqRounding8"=w218, "Duration8(s)"=w217, "Tones8"=w216, "RoundingVal8"=w215, "ApplyEQ"=w214, "Duration(s)"=w213, "CustomStimulusName"=w212, "Flatten Element Array"=w211, "sine waves"=w210, "Channel Out"=w209, "RatioVal6"=w208, "TabCtrl6"=w207, "Signal Type Name"=w206, "Help"="", "Channel Sel"=0 ("wave channel")) -> (w268:T1)
            }
            frame 4 {
              w275 = T7 {"StimulusType"="", "UseMLValArray"=[], "ML_axisArray"=[], "MLValLevelNameArray"=[], "Level(U)Array"=[], "Start(Stop)FreqArray"=[], "Start(Stop)AmpArray"=[], "StepResolutionArray"=[], "Unit_Array"=[], "DegValArray"=[], "DegUnitArray"=[], "Steps1"=0, "Cycle/step1(#)"=0, "Time/step1(s)"=0.0, "Transition1"=0.0, "SweepRate2"=0.0, "Freq3(Hz)"=0.0, "Steps3(#)"=0.0, "Cycles3(#)"=0, "StepSize3"=0.0, "wave time"="", "RMS_Value4"=0.0, "Peak_Value4"=0.0, "WavePath4"="", "RMS_unit4"="", "Peak_unit4"="", "wave Info"="", "dc_ctrl5_1"=0, "dc_ctrl5_2"=0, "dc_polar5"=0, "Max.Current"=0, "Steps5(#)"=0, "Time/Step5"=0.0, "Level5"=0.0, "StepsSize5Val"=0.0, "StepSize5Unit"="", "SweepType"=0, "Fixed/Ratio6"=0, "Transition6"=0.0, "Steps6(#)"=0.0, "Cycle/Steps6(#)"=0, "Time/Steps6(s)"=0.0, "Freq6(Hz)"=0.0, "Difference6(Hz)"=0.0, "Ratio6"="", "NoiseType7"=0, "Duration7(s)"=0.0, "MinFreq7(Hz)"=0.0, "MaxFreq7(Hz)"=0.0, "MinFreq8(Hz)"=0.0, "MaxFreq8(Hz)"=0.0, "FreqRounding8"=FALSE, "Duration8(s)"=0.0, "Tones8"=0.0, "RoundingVal8"=0.0, "ApplyEQ"=FALSE, "Duration(s)"=0.0, "CustomStimulusName "="", "Flatten Element Array"=[], "sine waves"=[], "Channel Out"=0, "RatioVal6"=0.0, "TabCtrl6"=enum."Master Tone", "Signal Type Name"="", "Help"="", "Channel Sel"=0}  # Stimulus4
              n42 = Unflatten From String(type=w275, binary string=w351) -> (value=w347:T7, error out=w349:errorcluster)  [unwired: 1 in, 3 out]
              n43 = Unbundle(w349) -> ("status"=w350:bool)  [unwired: 2 out]
              n44 = case shown="True" w350 {
                tunnel: w350 -> [_ w352]
                frame False {
                }
                frame True {
                  n45 = local write "Error?"(w352) -> ()
                }
              }
              n46 = Unbundle By Name(w347) -> ("StimulusType"=w345:string, "UseMLValArray"=w344:u16[], "ML_axisArray"=w343:u16[], "MLValLevelNameArray"=w339:string[], "Level(U)Array"=w340:dbl[], "Start(Stop)FreqArray"=w341:dbl[], "Start(Stop)AmpArray"=w342:dbl[], "DegValArray"=w338:dbl[], "DegUnitArray"=w337:string[], "Steps1"=w336:i32, "Cycle/step1(#)"=w335:u32, "Time/step1(s)"=w334:dbl, "Transition1"=w333:dbl, "SweepRate2"=w332:dbl, "Freq3(Hz)"=w331:dbl, "Steps3(#)"=w330:dbl, "Cycles3(#)"=w329:u32, "StepSize3"=w328:dbl, "wave time"=w327:string, "RMS_Value4"=w326:dbl, "Peak_Value4"=w325:dbl, "WavePath4"=w324:string, "RMS_unit4"=w323:string, "Peak_unit4"=w322:string, "wave Info"=w321:string, "dc_ctrl5_1"=w320:u16, "dc_ctrl5_2"=w319:u16, "dc_polar5"=w318:u16, "Max.Current"=w317:u16, "Steps5(#)"=w316:u32, "Time/Step5"=w315:dbl, "Level5"=w314:dbl, "StepsSize5Val"=w313:dbl, "StepSize5Unit"=w312:string, "SweepType"=w311:u16, "Fixed/Ratio6"=w310:u16, "Transition6"=w309:dbl, "Steps6(#)"=w308:dbl, "Cycle/Steps6(#)"=w307:u32, "Time/Steps6(s)"=w306:dbl, "Freq6(Hz)"=w305:dbl, "Difference6(Hz)"=w304:dbl, "Ratio6"=w303:string, "NoiseType7"=w302:u16, "Duration7(s)"=w301:dbl, "MinFreq7(Hz)"=w300:dbl, "MaxFreq7(Hz)"=w299:dbl, "MinFreq8(Hz)"=w298:dbl, "MaxFreq8(Hz)"=w297:dbl, "FreqRounding8"=w296:bool, "Duration8(s)"=w295:dbl, "Tones8"=w294:dbl, "RoundingVal8"=w293:dbl, "ApplyEQ"=w292:bool, "Duration(s)"=w291:dbl, "CustomStimulusName"=w290:string, "Flatten Element Array"=w289:string[], "sine waves"=w288:cluster{"freq":dbl, "ampl":dbl, "cycles":dbl}[], "Channel Out"=w287:i32, "RatioVal6"=w286:dbl, "TabCtrl6"=w285:enum32{"Master Tone", "Slave Tone"}, "Signal Type Name"=w284:string)  [unwired: 2 out]
              n47 = Initialize Array(u16 0 ("Unit"), 3 ("dimension size")) -> (w278:u16[])
              n48 = Initialize Array(u16 0 ("Unit"), 8 ("dimension size")) -> (w281:u16[])
              n49 = Bundle By Name(cluster=w348, "StimulusType"=w345, "UseMLValArray"=w344, "ML_axisArray"=w343, "MLValLevelNameArray"=w339, "Level(U)Array"=w340, "Start(Stop)FreqArray"=w341, "Start(Stop)AmpArray"=w342, "StepResolutionArray"=w278, "Unit_Array"=w281, "DegValArray"=w338, "DegUnitArray"=w337, "Steps1"=w336, "Cycle/step1(#)"=w335, "Time/step1(s)"=w334, "Transition1"=w333, "SweepRate2"=w332, "Freq3(Hz)"=w331, "Steps3(#)"=w330, "Cycles3(#)"=w329, "StepSize3"=w328, "wave time"=w327, "RMS_Value4"=w326, "Peak_Value4"=w325, "WavePath4"=w324, "RMS_unit4"=w323, "Peak_unit4"=w322, "wave Info"=w321, "dc_ctrl5_1"=w320, "dc_ctrl5_2"=w319, "dc_polar5"=w318, "Max.Current"=w317, "Steps5(#)"=w316, "Time/Step5"=w315, "Level5"=w314, "StepsSize5Val"=w313, "StepSize5Unit"=w312, "SweepType"=w311, "Fixed/Ratio6"=w310, "Transition6"=w309, "Steps6(#)"=w308, "Cycle/Steps6(#)"=w307, "Time/Steps6(s)"=w306, "Freq6(Hz)"=w305, "Difference6(Hz)"=w304, "Ratio6"=w303, "NoiseType7"=w302, "Duration7(s)"=w301, "MinFreq7(Hz)"=w300, "MaxFreq7(Hz)"=w299, "MinFreq8(Hz)"=w298, "MaxFreq8(Hz)"=w297, "FreqRounding8"=w296, "Duration8(s)"=w295, "Tones8"=w294, "RoundingVal8"=w293, "ApplyEQ"=w292, "Duration(s)"=w291, "CustomStimulusName"=w290, "Flatten Element Array"=w289, "sine waves"=w288, "Channel Out"=w287, "RatioVal6"=w286, "TabCtrl6"=w285, "Signal Type Name"=w284, "Help"="", "Channel Sel"=0 ("wave channel")) -> (w346:T1)
            }
            frame 5 {
              n50 = Unflatten From String(type=w354, binary string=w357) -> (value=w353:T1, error out=w355:errorcluster)  [unwired: 1 in, 3 out]
              n51 = Unbundle(w355) -> ("status"=w356:bool)  [unwired: 2 out]
              n52 = case shown="True" w356 {
                tunnel: w356 -> [_ w358]
                frame False {
                }
                frame True {
                  n53 = local write "Error?"(w358) -> ()
                }
              }
            }
            frame Default {
            }
          }
        }
      }
    }
    frame True {
      n54 = local write "Error?"(TRUE ("Error?")) -> ()
    }
  }
  "Stimulus" <- w2
  n55 = Bundle("substring"=w5, w6, "unsigned byte array[2]"=w7) -> (→"Header info":T8)  [unwired: 1 out]
